vi "AlliGator Compute Lifetime Simulation Histograms.vi"(0 "tau 1":dbl[](array[numeric]), 1 "Histogram Bin Size (tau)":dbl[unit], 2 "Histogram Bin Size (f1)":dbl, 5 "tau 2":dbl[](array[numeric]), 7 "a1":dbl[](array[numeric]), 11 "Error In":errorcluster, 12 "Percentiles to Keep (1, 99)":dbl[](array[numeric])=[99.0, 1.0]) -> (3 "Histograms":cluster{"Axis":dbl[], "Histogram":dbl[]}[](array[cluster]), 4 "Array Statistic (tau 1)":T1, 6 "Array Statistics (tau 2)":T1, 8 "Array Statistics (a1)":T1, 10 "Array of Scales":cluster{"X Scale":u32, "Y Scale":u32}[](array[cluster]), 13 "Plot Names":string[](array[string]), 14 "Message":string, 15 "Error Out":errorcluster)   [LabVIEW 2021, in "AlliGator Fit Method Benchmark.lvlib"]
doc: "Computes fitted parameter histograms and statistics."
uses:
  AlliGator Fit Method Benchmark.lvlib
  Arrays/Array Statistics.ctl
  Histograms/Linear Histogram Options.ctl
  Histograms/Histogram Bin Option.ctl
  Histograms/Histogram Bin Position.ctl
  5e0c3266-499e-46b2-80ef-c194e49f915b.vi
  9765538f-b151-4b8e-9b71-29b00fbc2fe4.vi
  8faa86fc-1a47-49e1-a18e-559db2184d30.vi
  6ac06ea2-d37e-43e0-baed-35fadc42c3ab.vi
  c2a6bf4c-2b36-4ed5-885f-cf0e0406484b.vi
  6045f332-e983-43bb-9ace-d0f5cff48457.vi
  dfa1e9a8-16d4-484e-b1d6-6a58a8855e91.vi
  5e0c3266-499e-46b2-80ef-c194e49f915b.vi/1ce800e1-bcd7-4855-83e2-66cab3687e54.vi
  9765538f-b151-4b8e-9b71-29b00fbc2fe4.vi/1ce800e1-bcd7-4855-83e2-66cab3687e54.vi
  8faa86fc-1a47-49e1-a18e-559db2184d30.vi/1ce800e1-bcd7-4855-83e2-66cab3687e54.vi
  6ac06ea2-d37e-43e0-baed-35fadc42c3ab.vi/e021cd17-e000-4244-b7f4-ec50548bdfcb.vi
  6ac06ea2-d37e-43e0-baed-35fadc42c3ab.vi/b1828c6e-eb0a-43e9-a724-8b596c52e435.vi
  6ac06ea2-d37e-43e0-baed-35fadc42c3ab.vi/7a6138ed-c001-4311-b538-9ba42ae7c7b1.vi
  6ac06ea2-d37e-43e0-baed-35fadc42c3ab.vi/52c6b4fa-501b-4af0-803b-8bab516ca5d3.vi
  6ac06ea2-d37e-43e0-baed-35fadc42c3ab.vi/d7237e10-35ab-4bcb-a0c6-4883c3f4c990.vi
  6ac06ea2-d37e-43e0-baed-35fadc42c3ab.vi/5fb5dd96-3b97-4592-ba56-58181c8e7105.vi
  6ac06ea2-d37e-43e0-baed-35fadc42c3ab.vi/8e13a849-a393-4484-9968-4af7b25c38d7.vi
  c2a6bf4c-2b36-4ed5-885f-cf0e0406484b.vi/e021cd17-e000-4244-b7f4-ec50548bdfcb.vi
  c2a6bf4c-2b36-4ed5-885f-cf0e0406484b.vi/b1828c6e-eb0a-43e9-a724-8b596c52e435.vi
  c2a6bf4c-2b36-4ed5-885f-cf0e0406484b.vi/7a6138ed-c001-4311-b538-9ba42ae7c7b1.vi
  c2a6bf4c-2b36-4ed5-885f-cf0e0406484b.vi/52c6b4fa-501b-4af0-803b-8bab516ca5d3.vi
  c2a6bf4c-2b36-4ed5-885f-cf0e0406484b.vi/d7237e10-35ab-4bcb-a0c6-4883c3f4c990.vi
  c2a6bf4c-2b36-4ed5-885f-cf0e0406484b.vi/5fb5dd96-3b97-4592-ba56-58181c8e7105.vi
  c2a6bf4c-2b36-4ed5-885f-cf0e0406484b.vi/8e13a849-a393-4484-9968-4af7b25c38d7.vi
  6045f332-e983-43bb-9ace-d0f5cff48457.vi/e021cd17-e000-4244-b7f4-ec50548bdfcb.vi
  6045f332-e983-43bb-9ace-d0f5cff48457.vi/b1828c6e-eb0a-43e9-a724-8b596c52e435.vi
  6045f332-e983-43bb-9ace-d0f5cff48457.vi/7a6138ed-c001-4311-b538-9ba42ae7c7b1.vi
  6045f332-e983-43bb-9ace-d0f5cff48457.vi/52c6b4fa-501b-4af0-803b-8bab516ca5d3.vi
  6045f332-e983-43bb-9ace-d0f5cff48457.vi/d7237e10-35ab-4bcb-a0c6-4883c3f4c990.vi
  6045f332-e983-43bb-9ace-d0f5cff48457.vi/5fb5dd96-3b97-4592-ba56-58181c8e7105.vi
  6045f332-e983-43bb-9ace-d0f5cff48457.vi/8e13a849-a393-4484-9968-4af7b25c38d7.vi
  dfa1e9a8-16d4-484e-b1d6-6a58a8855e91.vi/e021cd17-e000-4244-b7f4-ec50548bdfcb.vi
  dfa1e9a8-16d4-484e-b1d6-6a58a8855e91.vi/b1828c6e-eb0a-43e9-a724-8b596c52e435.vi
  dfa1e9a8-16d4-484e-b1d6-6a58a8855e91.vi/7a6138ed-c001-4311-b538-9ba42ae7c7b1.vi
  dfa1e9a8-16d4-484e-b1d6-6a58a8855e91.vi/52c6b4fa-501b-4af0-803b-8bab516ca5d3.vi
  dfa1e9a8-16d4-484e-b1d6-6a58a8855e91.vi/d7237e10-35ab-4bcb-a0c6-4883c3f4c990.vi
  dfa1e9a8-16d4-484e-b1d6-6a58a8855e91.vi/5fb5dd96-3b97-4592-ba56-58181c8e7105.vi
  dfa1e9a8-16d4-484e-b1d6-6a58a8855e91.vi/8e13a849-a393-4484-9968-4af7b25c38d7.vi
  Time/High Resolution Timing.vi
  <userlib>/_OpenG.lib/array/array.llb/Filter 1D Array__ogtk.vi
  <userlib>/_OpenG.lib/array/array.llb/Filter 1D Array (DBL)__ogtk.vi
  <userlib>/_OpenG.lib/array/array.llb/Delete Elements from Array__ogtk.vi
  <userlib>/_OpenG.lib/array/array.llb/Delete Elements from 1D Array (DBL)__ogtk.vi
  <vilib>/Utility/error.llb/Error Cluster From Error Code.vi
  Histograms/Histogram Window.lvlib
  Arrays/Arrays.lvlib
  Variant/Variant.lvlib
panel:
  # "see the AlliGator License on the block diagram (Ctrl+E or Window:Show Block Diagram)"
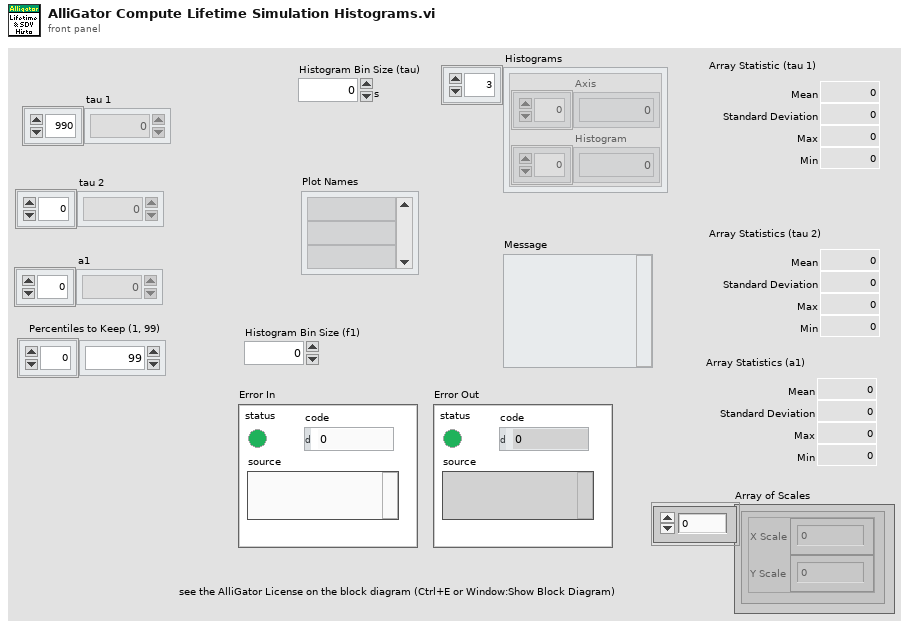
[diagram p1: front panel]
types:
  T1 = typedef "Arrays.lvlib/Array Statistics.ctl" = cluster{"Mean":dbl, "Standard Deviation":dbl, "Max":dbl, "Min":dbl}
  T2 = typedef "Histogram Window.lvlib/Linear Histogram Options.ctl" = cluster{"Bin Size":dbl, "Bin Number":i32, "Bin Option":T3, "Min Value":dbl, "Max Value":dbl, "Filter NaN & Infinite Values":bool, "Frequency Plot":bool, "Align Bins":bool, "Bin Location":T4, "Project Outside Values":bool, "Max Histogram Size":i32}
  T3 = typedef "Histogram Window.lvlib/Histogram Bin Option.ctl" = enum32{"Bin Number", "Bin Size"}
  T4 = typedef "Histogram Window.lvlib/Histogram Bin Position.ctl" = enum16{"Left", "Center", "Right"}
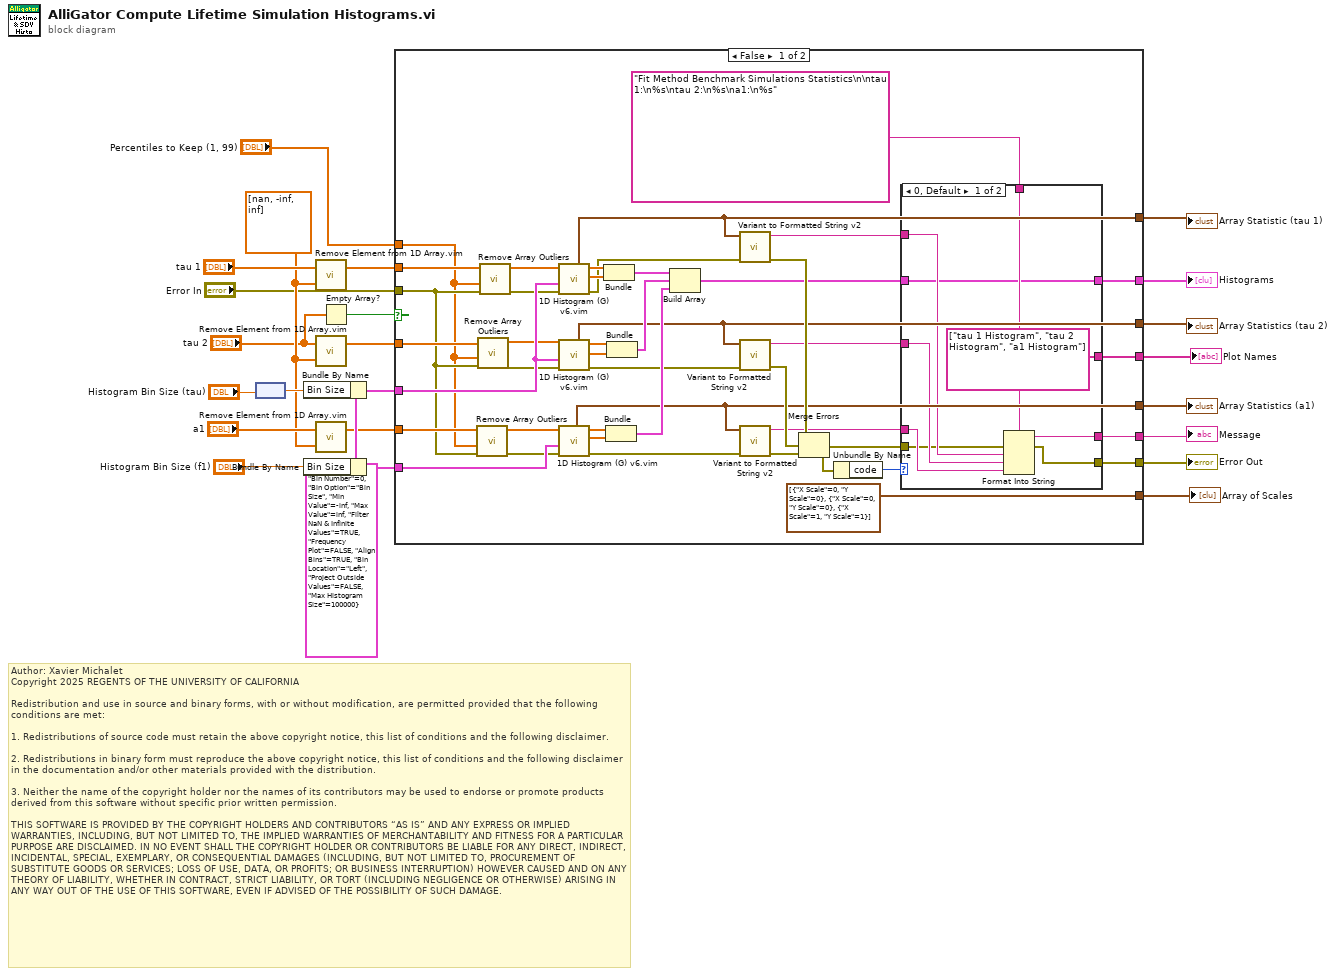
[diagram p0: block diagram]
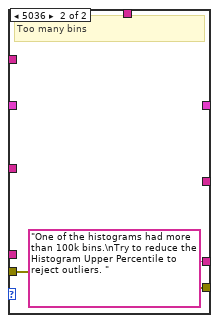
[diagram p2: hidden frame]
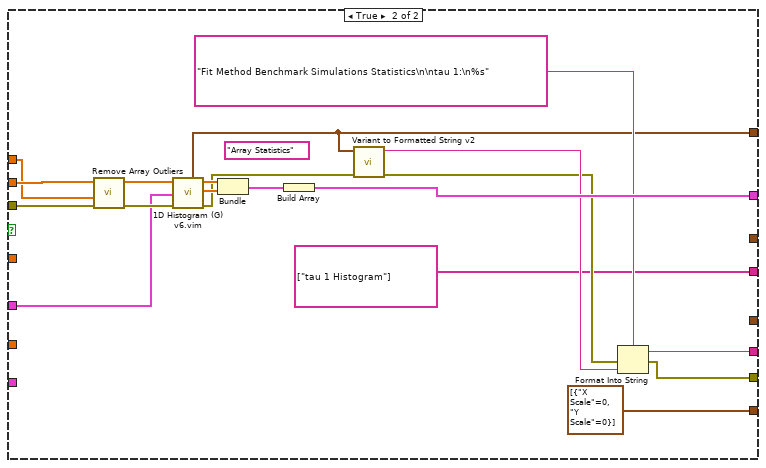
[diagram p3: hidden frame]
diagram:
  w16 = dbl[] [nan, -inf, inf] ("Element(s) to Remove")
  w23 = T2 {"Bin Size"=nan, "Bin Number"=0, "Bin Option"=enum."Bin Size", "Min Value"=-inf, "Max Value"=inf, "Filter NaN & Infinite Values"=TRUE, "Frequency Plot"=FALSE, "Align Bins"=TRUE, "Bin Location"=enum."Left", "Project Outside Values"=FALSE, "Max Histogram Size"=100000} ("Histogram Options")
  # "Author: Xavier Michalet\nCopyright 2025 REGENTS OF THE UNIVERSITY OF CALIFORNIA\n\nRedistribution and use in source and binary forms, with or without modification, are permitted provided that the following conditions are met:\n\n1. Redistributions of source code must retain the above copyright notice, this list of conditions and the following disclaimer.\n\n2. Redistributions in binary form must reproduce the above copyright notice, this list of conditions and the following disclaimer in the documentation and/or other materials provided with the distribution.\n\n3. Neither the name of the copyright holder nor the names of its contributors may be used to endorse or promote products derived from this software without specific prior written permission.\n\nTHIS SOFTWARE IS PROVIDED BY THE COPYRIGHT HOLDERS AND CONTRIBUTORS “AS IS” AND ANY EXPRESS OR IMPLIED WARRANTIES, INCLUDING, BUT NOT LIMITED TO, THE IMPLIED WARRANTIES OF MERCHANTABILITY AND FITNESS FOR A PARTICULAR PURPOSE ARE DISCLAIMED. IN NO EVENT SHALL THE COPYRIGHT HOLDER OR CONTRIBUTORS BE LIABLE FOR ANY DIRECT, INDIRECT, INCIDENTAL, SPECIAL, EXEMPLARY, OR CONSEQUENTIAL DAMAGES (INCLUDING, BUT NOT LIMITED TO, PROCUREMENT OF SUBSTITUTE GOODS OR SERVICES; LOSS OF USE, DATA, OR PROFITS; OR BUSINESS INTERRUPTION) HOWEVER CAUSED AND ON ANY THEORY OF LIABILITY, WHETHER IN CONTRACT, STRICT LIABILITY, OR TORT (INCLUDING NEGLIGENCE OR OTHERWISE) ARISING IN ANY WAY OUT OF THE USE OF THIS SOFTWARE, EVEN IF ADVISED OF THE POSSIBILITY OF SUCH DAMAGE."
  n1 = node("Histogram Bin Size (tau)") -> (w20:dbl)
  n2 = Bundle By Name(cluster=w23, "Bin Size"=w20) -> (w18:T2)
  n3 = Bundle By Name(cluster=w23, "Bin Size"="Histogram Bin Size (f1)") -> (w24:T2)
  n4 = call "Remove Element from 1D Array.vim"("Element(s) to Remove"=w16, "Input Array"="tau 1") -> ("Output Array"=w10:dbl[])  [unwired: 1 out]
  n5 = call "Remove Element from 1D Array.vim"("Element(s) to Remove"=w16, "Input Array"="tau 2") -> ("Output Array"=w9:dbl[])  [unwired: 1 out]
  n6 = call "Remove Element from 1D Array.vim"("Element(s) to Remove"=w16, "Input Array"="a1") -> ("Output Array"=w8:dbl[])  [unwired: 1 out]
  n7 = Empty Array?(array="tau 2") -> (empty?=w4:bool)
  n8 = case shown="False" w4 {
    tunnel: w24 -> [w67 _]
    tunnel: [w29 w97] -> w19
    tunnel: w18 -> [w57 w83]
    tunnel: [w56 w93] -> w15
    tunnel: [w55 w92] -> w14
    tunnel: [w26 _] -> w13
    tunnel: [w27 _] -> w12
    tunnel: [w28 w89] -> w11
    tunnel: w10 -> [w43 w82]
    tunnel: w9 -> [w41 _]
    tunnel: w8 -> [w38 _]
    tunnel: "Error In" -> [w35 w86]
    tunnel: "Percentiles to Keep (1, 99)" -> [w34 w81]
    tunnel: [w33 string[] ["tau 1 Histogram"] ("Plot Names")] -> w2
    tunnel: [cluster{"X Scale":u32, "Y Scale":u32}[] [{"X Scale"=0, "Y Scale"=0}, {"X Scale"=0, "Y Scale"=0}, {"X Scale"=1, "Y Scale"=1}] ("Array of Scales") cluster{"X Scale":u32, "Y Scale":u32}[] [{"X Scale"=0, "Y Scale"=0}] ("Array of Scales")] -> w1
    frame False {
      n9 = call "Remove Array Outliers.vi"("Error In"=w35, "Upper & Lower Percentile (100, 0)"=w34, "Array in"=w38) -> ("Error Out"=w36:errorcluster, "Array out"=w37:dbl[])  [unwired: 6 in, 1 out]
      n10 = call "Remove Array Outliers.vi"("Error In"=w35, "Upper & Lower Percentile (100, 0)"=w34, "Array in"=w41) -> ("Error Out"=w39:errorcluster, "Array out"=w40:dbl[])  [unwired: 6 in, 1 out]
      n11 = call "Remove Array Outliers.vi"("Error In"=w35, "Upper & Lower Percentile (100, 0)"=w34, "Array in"=w43) -> ("Error Out"=w42:errorcluster, "Array out"=w44:dbl[])  [unwired: 6 in, 1 out]
      n12 = call "1D Histogram (G) v6.vim"("Error In"=w42, "Histogram Options"=w57, "Array"=w44) -> ("Error Out"=w54:errorcluster, "Histogram"=w59:dbl[], "Axis"=w58:dbl[], "Array Statistics"=w28:T1)  [unwired: 2 in, 3 out]
      n13 = call "1D Histogram (G) v6.vim"("Error In"=w39, "Histogram Options"=w57, "Array"=w40) -> ("Error Out"=w53:errorcluster, "Histogram"=w61:dbl[], "Axis"=w60:dbl[], "Array Statistics"=w27:T1)  [unwired: 2 in, 3 out]
      n14 = call "1D Histogram (G) v6.vim"("Error In"=w36, "Histogram Options"=w67, "Array"=w37) -> ("Error Out"=w52:errorcluster, "Histogram"=w63:dbl[], "Axis"=w62:dbl[], "Array Statistics"=w26:T1)  [unwired: 2 in, 3 out]
      n15 = Bundle("Axis"=w58, "Histogram"=w59) -> (w64:cluster{"Axis":dbl[], "Histogram":dbl[]})  [unwired: 1 in]
      n16 = Bundle("Axis"=w62, "Histogram"=w63) -> (w66:cluster{"Axis":dbl[], "Histogram":dbl[]})  [unwired: 1 in]
      n17 = Bundle("Axis"=w60, "Histogram"=w61) -> (w65:cluster{"Axis":dbl[], "Histogram":dbl[]})  [unwired: 1 in]
      n18 = Build Array(w64, w65, w66) -> (w30:cluster{"Axis":dbl[], "Histogram":dbl[]}[])
      n19 = call "Variant to Formatted String v2.vi"("error in (no error)"=w54, "Anything"=w28) -> ("error out"=w51:errorcluster, "String"=w48:string)  [unwired: 8 in]
      n20 = call "Variant to Formatted String v2.vi"("error in (no error)"=w53, "Anything"=w27) -> ("error out"=w50:errorcluster, "String"=w47:string)  [unwired: 8 in]
      n21 = call "Variant to Formatted String v2.vi"("error in (no error)"=w52, "Anything"=w26) -> ("error out"=w49:errorcluster, "String"=w46:string)  [unwired: 8 in]
      n22 = Merge Errors(w51, w50, w49) -> (w32:errorcluster)
      n23 = Unbundle By Name(w32) -> ("code"=w31:i32)
      n24 = case shown="0, Default" w31 {
        tunnel: [w76 "One of the histograms had more than 100k bins.\nTry to reduce the Histogram Upper Percentile to reject outliers. "] -> w56
        tunnel: [w75 w78] -> w55
        tunnel: w48 -> [w74 _]
        tunnel: w47 -> [w73 _]
        tunnel: w46 -> [w72 _]
        tunnel: "Fit Method Benchmark Simulations Statistics\n\ntau 1:\n%s\ntau 2:\n%s\na1:\n%s" ("format string") -> [w71 _]
        tunnel: [string[] ["tau 1 Histogram", "tau 2 Histogram", "a1 Histogram"] ("Plot Names") _] -> w33
        tunnel: w32 -> [w69 w78]
        tunnel: w30 -> [w68 _]
        tunnel: [w68 _] -> w29
        frame 0, Default {
          n25 = Format Into String(format string=w71, error in=w69, w74, w73, w72) -> (resulting string=w76:string, error out=w75:errorcluster)  [unwired: 1 in]
        }
        frame 5036 {
          # "Too many bins"
        }
      }
    }
    frame True {
      (unwired) "Array Statistics" ("Label")
      n26 = call "Remove Array Outliers.vi"("Error In"=w86, "Upper & Lower Percentile (100, 0)"=w81, "Array in"=w82) -> ("Error Out"=w87:errorcluster, "Array out"=w88:dbl[])  [unwired: 6 in, 1 out]
      n27 = call "1D Histogram (G) v6.vim"("Error In"=w87, "Histogram Options"=w83, "Array"=w88) -> ("Error Out"=w91:errorcluster, "Histogram"=w95:dbl[], "Axis"=w94:dbl[], "Array Statistics"=w89:T1)  [unwired: 2 in, 3 out]
      n28 = Bundle("Axis"=w94, "Histogram"=w95) -> (w96:cluster{"Axis":dbl[], "Histogram":dbl[]})  [unwired: 1 in]
      n29 = Build Array(w96) -> (w97:cluster{"Axis":dbl[], "Histogram":dbl[]}[])
      n30 = call "Variant to Formatted String v2.vi"("error in (no error)"=w91, "Anything"=w89) -> ("error out"=w84:errorcluster, "String"=w85:string)  [unwired: 8 in]
      n31 = Format Into String(format string="Fit Method Benchmark Simulations Statistics\n\ntau 1:\n%s", error in=w84, w85) -> (resulting string=w93:string, error out=w92:errorcluster)  [unwired: 1 in]
    }
  }
  "Histograms" <- w19
  "Array Statistics (tau 2)" <- w12
  "Array Statistic (tau 1)" <- w11
  "Array Statistics (a1)" <- w13
  "Error Out" <- w14
  "Message" <- w15
  "Plot Names" <- w2
  "Array of Scales" <- w1
